vi "Plot Data.vi"(8 "error in (no error)":errorcluster, 11 "GUI In":refnum<class "Calibration UI.lvclass">) -> (0 "error out":errorcluster, 1 "Fit Data":T1(array[cluster]), 2 "Plot Data":cluster{dbl[], "Upper Bound":dbl[]}[][](array[cluster]), 5 "Data Available?":bool)   [LabVIEW 2015, in "Calibration UI.lvclass"]
uses:
  Calibration UI.lvclass
  Calibration UI.lvclass/Calibration UI.ctl
  Calibration/State data/State Data.lvclass/State Data.ctl
  Calibration/State data/Read Extinction.vi
  Calibration/State data/Read IA.vi
  <vilib>/Analysis/6fits.llb/Prediction Interval (Linear).vi
  <vilib>/Analysis/NI_AALPro.lvlib
  Calibration/State data/State Data.lvclass
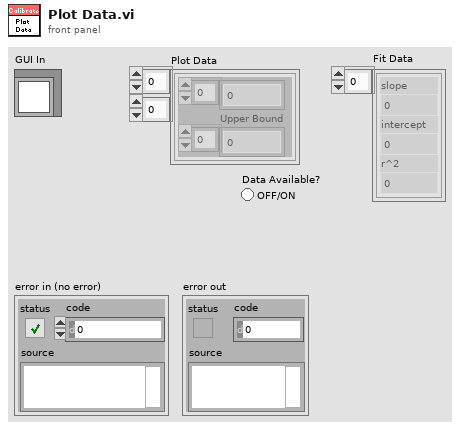
[diagram p1: front panel]
types:
  T1 = cluster{"slope":dbl, "intercept":dbl, "r^2":dbl}[]
  T2 = cluster{"Stored State":refnum<class "State Data.lvclass">[], "pointer to data":i32}
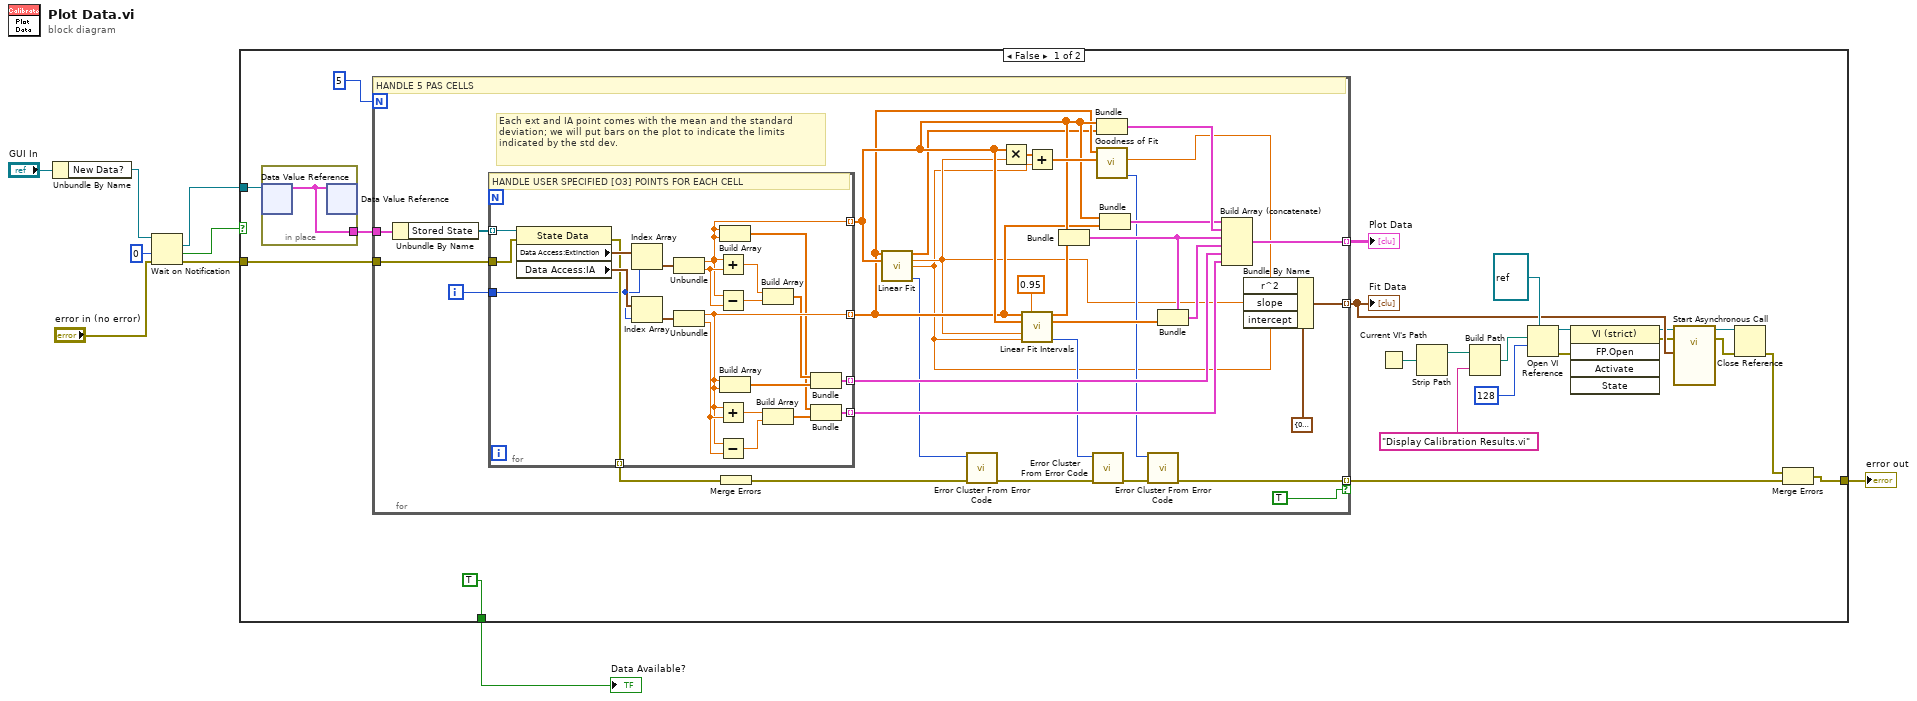
[diagram p0: block diagram]
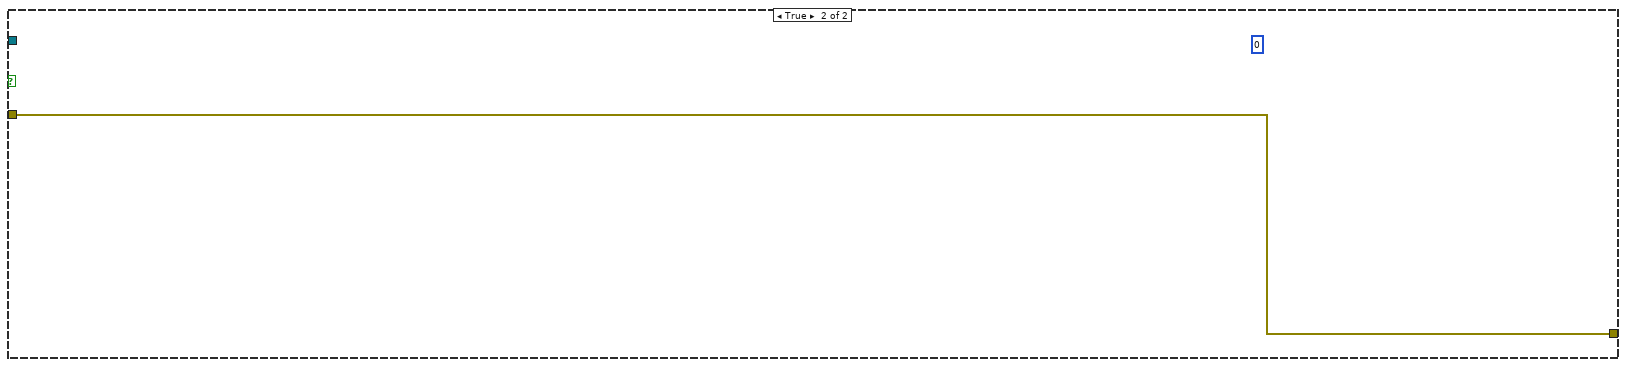
[diagram p2: hidden frame]
diagram:
  n1 = Unbundle By Name("GUI In") -> ("New Data?"=w7:refnum<notifier>)
  n2 = Wait on Notification(notifier=w7, timeout in ms (-1)=0, error in (no error)="error in (no error)") -> (notification=w6:refnum<data-value>, timed out?=w3:bool, error out=w4:errorcluster)  [unwired: 1 in, 1 out]
  n3 = case shown="False" w3 {
    tunnel: w4 -> [w31 w88]
    tunnel: [w27 w88] -> w1
    tunnel: w6 -> [w30 _]
    tunnel: [TRUE _] -> w2
    frame False {
      n4 = in-place {
        in-place-border: [w87] -> w26
        n5 = in-place-dvr #1(w30) -> (w87:T2)  [unwired: 1 out]
        n6 = in-place-dvr #1(w87) -> ()  [unwired: 2 out]
      }
      n7 = for {
        N: 5 -> [_]
        tunnel: w26 -> [w54]
        tunnel: w31 -> [w48]
        tunnel: [w39] -> w28 mode=indexing if=TRUE
        tunnel: [w37] -> w24 mode=indexing
        tunnel: [w34] -> w17 mode=indexing
        i -> [w38]
        # "Each ext and IA point comes with the mean and the standard deviation; we will put bars on the plot to indicate the limits indicated by the std dev."
        # "HANDLE 5 PAS CELLS"
        n8 = Unbundle By Name(w54) -> ("Stored State"=w55:refnum<class "State Data.lvclass">[])
        n9 = for {
          tunnel: w55 -> [w86] mode=indexing
          tunnel: [w77] -> w62 mode=indexing
          tunnel: [w81] -> w61 mode=indexing
          tunnel: [w78] -> w52 mode=indexing
          tunnel: [w72] -> w53 mode=indexing
          tunnel: w48 -> [w67]
          tunnel: [w66] -> w44 mode=indexing
          tunnel: w38 -> [w65]
          # "HANDLE USER SPECIFIED [O3] POINTS FOR EACH CELL"
          n10 = property class="State Data"(reference=w86, error in=w67) -> (error out=w66:errorcluster, "Data Access:Extinction"=w71:cluster{"Mean":dbl, "Error":dbl}[], "Data Access:IA"=w69:cluster{"Mean":dbl, "Error":dbl}[])  [unwired: 1 out]
          n11 = Index Array(array=w71, index=w65) -> (element=w70:cluster{"Mean":dbl, "Error":dbl})
          n12 = Index Array(array=w69, index=w65) -> (element=w68:cluster{"Mean":dbl, "Error":dbl})
          n13 = Unbundle(w70) -> ("Mean"=w77:dbl, "Error"=w85:dbl)
          n14 = Unbundle(w68) -> ("Mean"=w81:dbl, "Error"=w84:dbl)
          n15 = Add(x=w77, y=w85) -> (x+y=w82:dbl)
          n16 = Subtract(x=w77, y=w85) -> (x-y=w83:dbl)
          n17 = Add(x=w81, y=w84) -> (x+y=w76:dbl)
          n18 = Subtract(x=w81, y=w84) -> (x-y=w75:dbl)
          n19 = Build Array(w77, w77) -> (w74:dbl[])
          n20 = Build Array(w81, w81) -> (w80:dbl[])
          n21 = Build Array(w82, w83) -> (w79:dbl[])
          n22 = Build Array(w76, w75) -> (w73:dbl[])
          n23 = Bundle(w79, w80) -> (w78:cluster{dbl[], dbl[]})  [unwired: 1 in]
          n24 = Bundle(w74, w73) -> (w72:cluster{dbl[], dbl[]})  [unwired: 1 in]
        }
        n25 = Merge Errors(w44) -> (w43:errorcluster)
        n26 = call <vilib>:"Linear Fit.vi"("Y"=w61, "X"=w62) -> ("Best Linear Fit"=w49:dbl[], "slope"=w36:dbl, "intercept"=w35:dbl, "error"=w46:i32)  [unwired: 9 in, 1 out]
        n27 = call <vilib>:"Error Cluster From Error Code.vi"("error in (no error)"=w43, "error code (0)"=w46) -> ("error out"=w45:errorcluster)  [unwired: 7 in]
        n28 = Multiply(x=w62, y=w36) -> (x*y=w63:dbl[])
        n29 = call-poly <vilib>:"Linear Fit Intervals.vi"("Y"=w61, "confidence level"=0.95, "X"=w62, "slope"=w36, "intercept"=w35) -> ("Upper Bound"=w57:dbl[], "Lower Bound"=w58:dbl[], "error"=w47:i32)  [unwired: 8 in]
        n30 = Add(x=w63, y=w35) -> (x+y=w64:dbl[])
        n31 = Bundle(w62, "Upper Bound"=w57) -> (w59:cluster{dbl[], "Upper Bound":dbl[]})  [unwired: 1 in]
        n32 = call <vilib>:"Error Cluster From Error Code.vi"("error in (no error)"=w45, "error code (0)"=w47) -> ("error out"=w40:errorcluster)  [unwired: 7 in]
        n33 = Bundle(w62, "Best Linear Fit"=w49) -> (w51:cluster{dbl[], "Best Linear Fit":dbl[]})  [unwired: 1 in]
        n34 = call <vilib>:"Goodness of Fit.vi"("Best Fit"=w64, "Y"=w61) -> ("error"=w41:i32, "R-square"=w32:dbl)  [unwired: 6 in, 2 out]
        n35 = Bundle(w62, w61) -> (w50:cluster{dbl[], dbl[]})  [unwired: 1 in]
        n36 = call <vilib>:"Error Cluster From Error Code.vi"("error in (no error)"=w40, "error code (0)"=w41) -> ("error out"=w39:errorcluster)  [unwired: 7 in]
        n37 = Bundle(cluster=w59, "Upper Bound"=w58) -> (w60:cluster{dbl[], "Upper Bound":dbl[]})  [unwired: 1 in]
        n38 = Build Array (concatenate)(w50, w51, w59, w60, w52, w53) -> (w37:cluster{dbl[], "Upper Bound":dbl[]}[])
        n39 = Bundle By Name(cluster=cluster{"slope":dbl, "intercept":dbl, "r^2":dbl} {"slope"=0.0, "intercept"=0.0, "r^2"=0.0} ("Linear Fit Data"), "r^2"=w32, "slope"=w36, "intercept"=w35) -> (w34:cluster{"slope":dbl, "intercept":dbl, "r^2":dbl})
      }
      "Plot Data" <- w24
      "Fit Data" <- w17
      n40 = Current VI's Path() -> (path=w22:path)
      n41 = Strip Path(path=w22) -> (stripped path=w21:path)  [unwired: 1 out]
      n42 = Build Path(base path=w21, name or relative path="Display Calibration Results.vi") -> (appended path=w19:path)
      n43 = Open VI Reference(type specifier VI Refnum (for type only)=refnum<vi> refnum, vi path=w19, options=128) -> (vi reference=w13:refnum<vi>, error out=w11:errorcluster)  [unwired: 3 in]
      n44 = invoke class="VI (strict)" method="FP.Open"(reference=w13, error in=w11) -> (reference out=w12:refnum<vi>, error out=w10:errorcluster)  [unwired: 3 in, 3 out]
      n45 = call-by-ref "Start Asynchronous Call"(reference=w12, error in=w10, "Fit Data"=w17) -> (reference out=w16:refnum<vi>, error out=w15:errorcluster)  [unwired: 11 in]
      n46 = Close Reference(reference=w16, error in (no error)=w15) -> (error out=w14:errorcluster)
      n47 = Merge Errors(w14, w28) -> (w27:errorcluster)
    }
    frame True {
      (unwired) 0 ("error")
    }
  }
  "error out" <- w1
  "Data Available?" <- w2
